vi "8-Tap 8-bit Camera with DRAM Modified (FPGA).vi"() -> ()   [LabVIEW 2013]
doc: "This is the FPGA VI for the 10-Tap 8-Bit Camera with DRAM example. This example demonstrates how to acquire images from a 10-tap, 8-bit, extended configuration, Camera Link camera and transfer the images to the host. This example supports area scan and line scan cameras for both continuous and finite acquisitions.\n\nThis example also demonstrates the use of DRAM as a frame buffer for very high speed acquisitions. Data packing and flow-control are also employed to maximize use of the available DRAM and FIFOs in terms of both memory space and performance.\n\nAdditionally, the example demonstrates the serial server, which allows third-party camera configuration utilities to communicate with the camera using the Camera Link serial interface while this VI is running."
uses:
  Common/CL Signal Mapping.ctl
  Common/CL Configuration.ctl
  <vilib>/Platform/TimedLoop/XDataNode/timing_clust.ctl
  <vilib>/Platform/TimedLoop/XDataNode/nitl_modes.ctl
  <vilib>/Platform/TimedLoop/XDataNode/wakeup.ctl
  <vilib>/rvi/Emulation/niFpgaSctlEmulationGetInTimedLoop.vi
  <vilib>/rvi/Emulation/niFpgaEmulationReportErrorSimple.vi
  <vilib>/rvi/eio/common/nirviEmuTemplateMethod_errors.vi
  <vilib>/rvi/Emulation/niFpgaGetClockAttributes.vi
  <vilib>/rvi/Emulation/niFpgaCriticalErrorInLSC.vi
  Common/CL Data to Pixels/8 Tap 8-Bit.vi
  <vilib>/rvi/FIFO/Fifo_Resource/nirvififoEmulationWriteFpgaImpl.vi
  <vilib>/rvi/DataTransferAndStorage/Container/Common/niFpgaContainerGetUniqueNameForEmu.vi
  <vilib>/rvi/FIFO/Fifo_Resource/nirvififoEmulationGetNumberOfElementsToReadFpgaImpl.vi
  <vilib>/rvi/FIFO/Fifo_Resource/nirvififoEmulationReadFpgaImpl.vi
  <vilib>/rvi/interface/RandomDataEmulation/nirviRandomDataFPGAFIFO.vi
  <vilib>/rvi/interface/RandomDataEmulation/niFpgaRandomDataHandleErrors.vi
  <vilib>/rvi/Emulation/niFpgaProcessEmulError.vi
  <vilib>/Platform/TimedLoop/XDataNode/XDataNode.xnode
  <vilib>/eio/EIONode/EIONode.xnode
  <vilib>/rvi/DataTransferAndStorage/Container/XNode/niFpgaContainer.xnode
  <vilib>/rvi/FIFO/Fifo_Resource/nirvififoEmulationWrite.vi
  <vilib>/rvi/FIFO/Fifo_Resource/nirvififoEmulationGetNumberOfElementsToRead.vi
  <vilib>/rvi/FIFO/Fifo_Resource/nirvififoEmulationRead.vi
  <vilib>/rvi/interface/RandomDataEmulation/nirviRandomDataFpgaReadWriteTemplate.vi
  <vilib>/Platform/TimedLoop/XDataNode/XDNodeRunTimeDep.lvlib
panel:
  out "DMA Full?":bool
  in  "CL Config.Configuration":T1=enum."Full"
  in  "CL Config.Signal Mapping":T2
  in  "CL Config.Line Scan":bool
  in  "CL Config.DVAL Active High":bool=TRUE
  in  "CL Config.LVAL Active High":bool=TRUE
  in  "CL Config.FVAL Active High":bool=TRUE
  in  "CL Config.Spare Active High":bool=TRUE
  in  "Acq Control.Line Scan Height":u32
  in  "Acq Control.Frames To Acq":u32
  in  "Acq Control.Acquire":bool
  in  "Acq Control.Cancel Acq":bool
  in  "Acq Control.Ignore DVAL":bool
  in  "Acq Control.Initialize":bool
  out "Acq Status.Acq In Progress":bool
  out "Acq Status.Clocks Per Line":u32
  out "Acq Status.Frames Acq'd":u32
  out "Acq Status.Lines Per Frame":u32
  out "Acq Status.DMA Write Timeout":bool
  out "Acq Status.Initialized":bool
  in  "UART.Baud Rate":u8
  in  "UART.Transmit":bool
  in  "UART.Tx Data":u8[](array[numeric])=[0, 0, 0, 0, 0, 0, 0, 0, 0, 0] format="%02x"
  in  "UART.Set Baud Rate":bool
  in  "UART.Byte Mode":bool=TRUE
  out "UART.Rx Ready":bool
  out "UART.Break Indicator":bool
  out "UART.Framing Error":bool
  out "UART.Overrun Error":bool
  out "UART.Tx Ready":bool
  out "UART.Rx Data":u8 format="%02x"
  in  "UART.Receive":bool
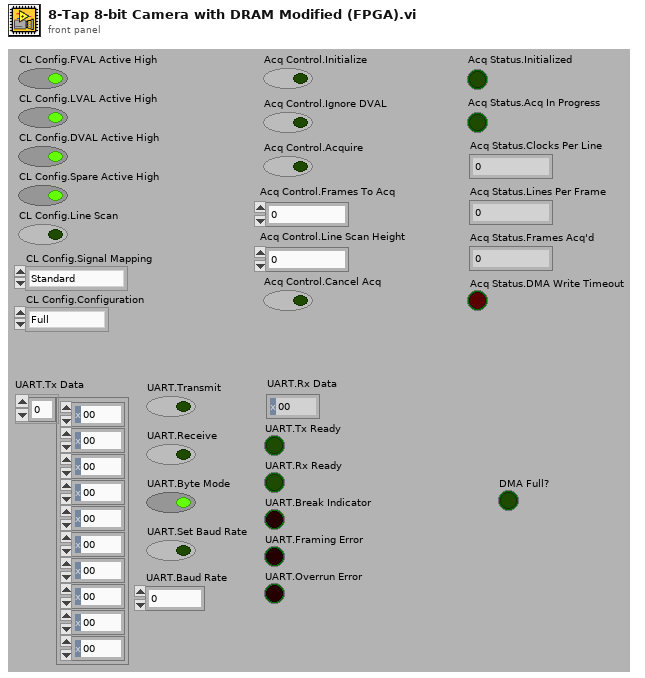
[diagram p1: front panel]
types:
  T1 = typedef "CL Configuration.ctl" = enum8{"Base", "Medium", "Full"}
  T2 = typedef "CL Signal Mapping.ctl" = enum8{"Standard", "Basler 10-tap", "Vosskühler 10-tap"}
  T3 = typedef "XDNodeRunTimeDep.lvlib/timing_clust.ctl" = cluster{"Expected End [f-1]":u64, "Actual End [f-1]":u64, "Finished Late? [f-1]":bool, "Expected End [i-1]":u64, "Actual End [i-1]":u64, "Finished Late? [i-1]":bool, "Expected Start [i]":u64, "Actual Start [i]":u64, "Expected Start [f]":u64, "Actual Start [f]":u64, "Source Name":string, "Structure Name":string, "Period":i64, "Deadline":i64, "Offset":i64, "Start":i64, "Priority":i32, "Timeout":i32, "Mode":T4, "Wakeup Reason":T5, "Error":errorcluster, "Source Type":string, "Secondary Source Type":string, "Global End Time":u64, "Global Start Time":u64, "Frame Duration":u64, "Iteration Duration":u64, "Assigned CPU":i32, "I/O Scan Engine Mode":u32}
  T4 = typedef "XDNodeRunTimeDep.lvlib/nitl_modes.ctl" = enum32{"No Change", "Process missed periods, maintain original phase", "Discard missed periods, maintain original phase", "Process missed periods, ignore original phase", "Discard missed periods, ignore original phase"}
  T5 = typedef "XDNodeRunTimeDep.lvlib/wakeup.ctl" = enum32{"Normal", "Aborted", "Asynchronous wakeup", "Timing source error", "Timed loop error", "Timeout"}
  T6 = cluster{"Enables Valid":bool, "Frame Valid":bool, "Line Valid":bool, "Data Valid":bool}
  T7 = cluster{"Pixel 0":u8, "Pixel 1":u8, "Pixel 2":u8, "Pixel 3":u8, "Pixel 4":u8, "Pixel 5":u8, "Pixel 6":u8, "Pixel 7":u8}
  T8 = cluster{"Tx Data":u8[], "Transmit":bool, "Receive":bool, "Byte Mode":bool, "Set Baud Rate":bool, "Baud Rate":u8}
  T9 = cluster{"Rx Data":u8, "Turn Off Transmit":bool, "Turn Off Receive":bool, "Turn Off Set Baud Rate":bool, "Tx Ready":bool, "Rx Ready":bool, "Break Indicator":bool, "Framing Error":bool, "Overrun Error":bool}
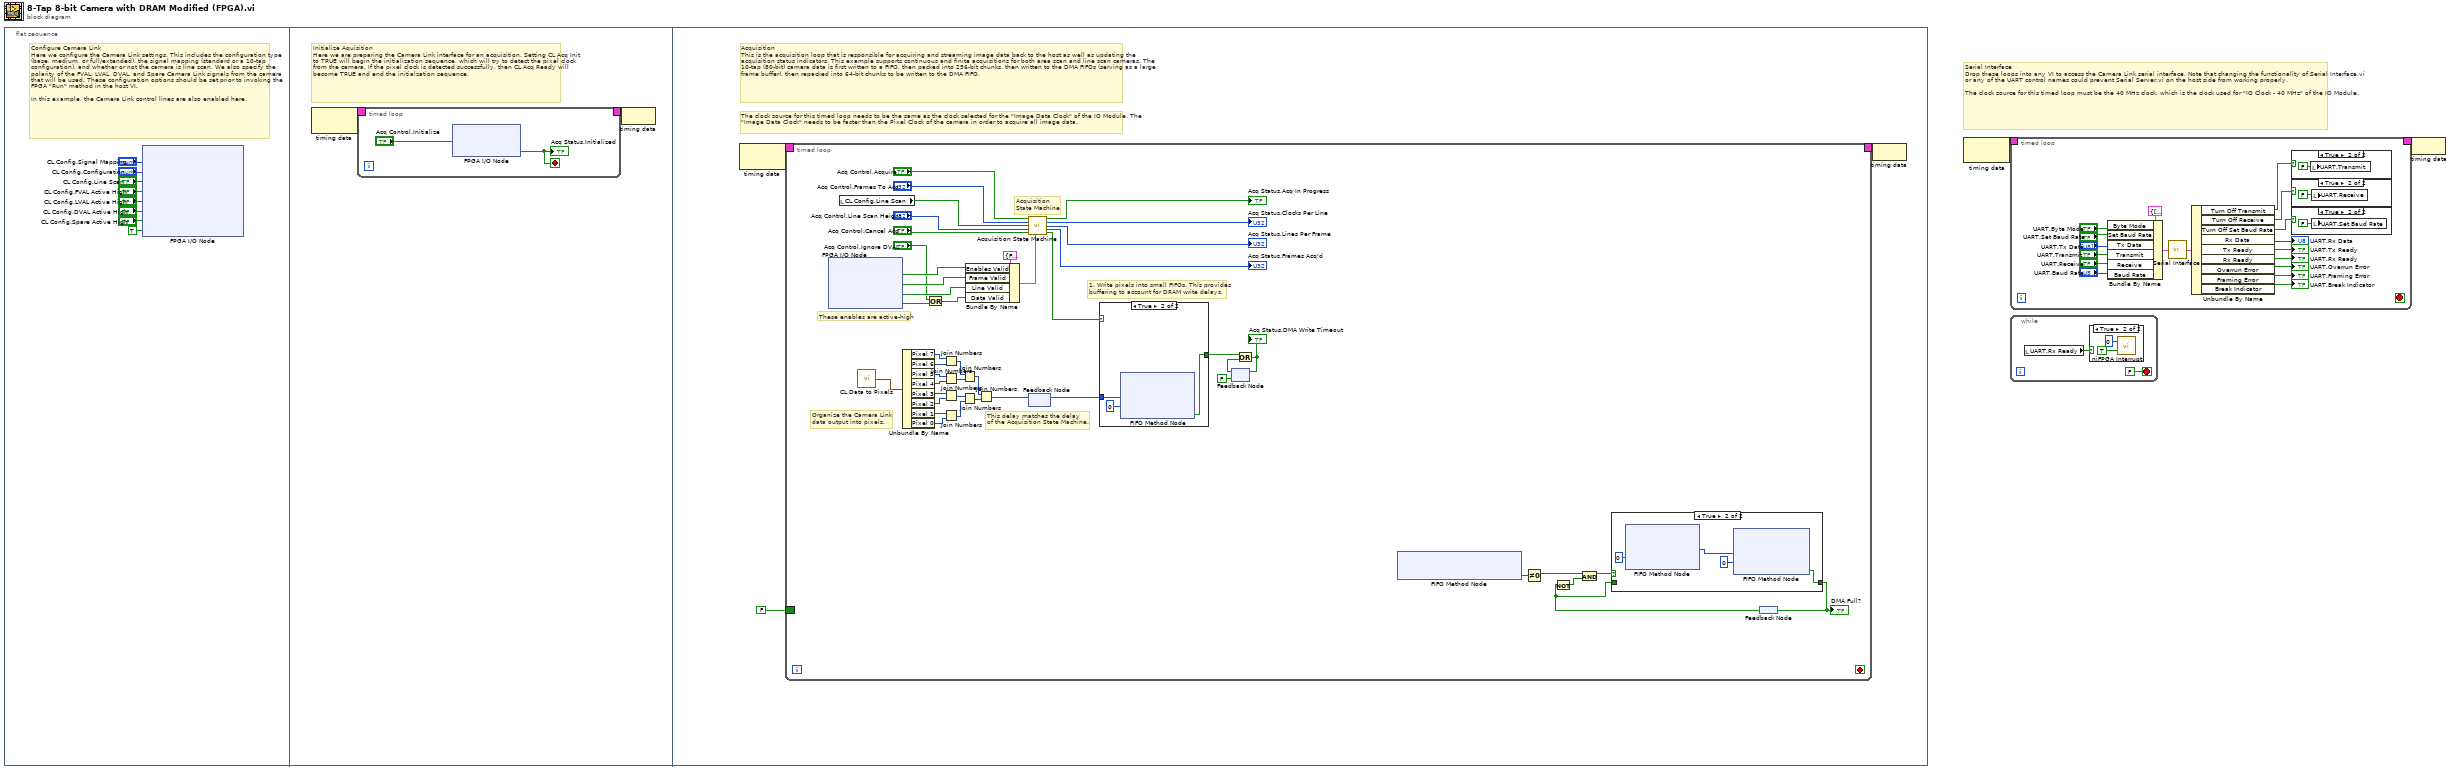
[diagram p0: block diagram]
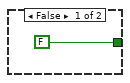
[diagram p7: hidden frame]
diagram:
  # "Serial Interface\nDrop these loops into any VI to access the Camera Link serial interface. Note that changing the functionality of Serial Interface.vi or any of the UART control names could prevent Serial Server.vi on the host side from working properly.\n\nThe clock source for this timed loop must be the 40 MHz clock, which is the clock used for \"IO Clock - 40 MHz\" of the IO Module."
  n1 = flat-sequence {
    frame #0 {
      # "Configure Camera Link\nHere we configure the Camera Link settings. This includes the configuration type (base, medium, or full/extended), the signal mapping (standard or a 10-tap configuration), and whether or not the camera is line scan. We also specify the polarity of the FVAL, LVAL, DVAL, and Spare Camera Link signals from the camera that will be used. These configuration options should be set prior to invoking the FPGA \"Run\" method in the host VI.\n\nIn this example, the Camera Link control lines are also enabled here."
      n2 = xnode "FPGA I/O Node"("CL Set Signal Mapping"="CL Config.Signal Mapping", "CL Set Configuration"="CL Config.Configuration", "CL Set Line Scan"="CL Config.Line Scan", "CL Set FVAL Active High"="CL Config.FVAL Active High", "CL Set LVAL Active High"="CL Config.LVAL Active High", "CL Set DVAL Active High"="CL Config.DVAL Active High", "CL Set Spare Active High"="CL Config.Spare Active High", "CL Control Enable"=TRUE ("IO Module\\CL Control Enable")) -> ()  [unwired: 8 in, 8 out]
    }
    frame #1 {
      # "Initialize Aquisition\nHere we are preparing the Camera Link interface for an acquisition. Setting CL Acq Init to TRUE will begin the initialization sequence, which will try to detect the pixel clock from the camera. If the pixel clock is detected successfully, then CL Acq Ready will become TRUE and end the initialzation sequence."
      n3 = node-c288() -> (w12:T3)  [unwired: 1 out]
      n4 = timed-loop {
        timing: w12 -> [_]
        timing-out: [_] -> w11
        stop <- w13 stop-if-true
        n5 = xnode "FPGA I/O Node"("CL Acq Init"="Acq Control.Initialize") -> ("CL Acq Ready"=w13:bool)  [unwired: 2 in, 2 out]
        "Acq Status.Initialized" <- w13
      }
      n6 = node-c288(w11) -> ()
    }
    frame #2 {
      # "The clock source for this timed loop needs to be the same as the clock selected for the \"Image Data Clock\" of the IO Module. The \"Image Data Clock\" needs to be faster than the Pixel Clock of the camera in order to acquire all image data."
      # "Acquisition\nThis is the acquisition loop that is responsible for acquiring and streaming image data back to the host as well as updating the acquisition status indicators. This example supports continuous and finite acquisitions for both area scan and line scan cameras. The 10-tap (80-bit) camera data is first written to a FIFO, then packed into 256-bit chunks, then written to the DMA FIFOs (serving as a large frame buffer), then repacked into 64-bit chunks to be written to the DMA FIFO."
      n7 = node-c288() -> (w21:T3)  [unwired: 1 in]
      n8 = timed-loop {
        timing: w21 -> [_]
        timing-out: [_] -> w20
        border: FALSE ("Timed Out?") -> [_]
        stop <- _ stop-if-true
        # "1. Write pixels into small FIFOs. This provides\nbuffering to account for DRAM write delays."
        # "Organize the Camera Link\ndata output into pixels."
        # "These enables are active-high"
        # "This delay matches the delay\nof the Acquisition State Machine."
        # "Acquisition\nState Machine"
        n9 = xnode "FPGA I/O Node"() -> ("CL Output Valid"=w52:bool, "CL Frame Valid"=w51:bool, "CL Line Valid"=w50:bool, "CL Data Valid"=w47:bool)  [unwired: 4 in, 4 out]
        n10 = local read "CL Config.Line Scan"() -> (w44:bool)
        n11 = call-poly "CL Data to Pixels.vi"() -> ("Pixels"=w66:T7)  [unwired: 1 in]
        n12 = Unbundle By Name(w66) -> ("Pixel 7"=w42:u8, "Pixel 6"=w41:u8, "Pixel 5"=w40:u8, "Pixel 4"=w39:u8, "Pixel 3"=w38:u8, "Pixel 2"=w37:u8, "Pixel 1"=w36:u8, "Pixel 0"=w35:u8)
        n13 = Or(x="Acq Control.Ignore DVAL", y=w47) -> (x .or. y?=w46:bool)
        n14 = Join Numbers(hi=w42, lo=w41) -> ((hi.lo)=w33:u16)
        n15 = Join Numbers(hi=w40, lo=w39) -> ((hi.lo)=w32:u16)
        n16 = Join Numbers(hi=w38, lo=w37) -> ((hi.lo)=w31:u16)
        n17 = Join Numbers(hi=w36, lo=w35) -> ((hi.lo)=w34:u16)
        n18 = Join Numbers(hi=w33, lo=w32) -> ((hi.lo)=w30:u32)
        n19 = Join Numbers(hi=w31, lo=w34) -> ((hi.lo)=w29:u32)
        n20 = Bundle By Name(cluster=T6 {"Enables Valid"=FALSE, "Frame Valid"=FALSE, "Line Valid"=FALSE, "Data Valid"=FALSE} ("Enables"), "Enables Valid"=w52, "Frame Valid"=w51, "Line Valid"=w50, "Data Valid"=w46) -> (w49:T6)
        n21 = Join Numbers(hi=w30, lo=w29) -> ((hi.lo)=w28:u64)
        n22 = call "Acquisition State Machine.vi"("Acquire"="Acq Control.Acquire", "Frames to Acquire"="Acq Control.Frames To Acq", "Line Scan"=w44, "Line Scan Height"="Acq Control.Line Scan Height", "Cancel Acq"="Acq Control.Cancel Acq", "Enables"=w49) -> ("Acq In Progress"=→"Acq Status.Acq In Progress":bool, "Num Clocks Per Line"=→"Acq Status.Clocks Per Line":u32, "Num Lines Per Frame"=→"Acq Status.Lines Per Frame":u32, "Num Frames Acq'd"=→"Acq Status.Frames Acq'd":u32, "Capture Cycle"=w64:bool)  [unwired: 4 in, 1 out]
        n23 = feedback-in #1(w28) -> ()
        n24 = feedback #1() -> (w65:u64)  [unwired: 1 in]
        n25 = case shown="True" w64 {
          tunnel: [FALSE ("Timed Out?") w74] -> w62
          tunnel: w65 -> [_ w75]
          frame False {
          }
          frame True {
            n26 = xnode ("FIFO Method Node")("Element"=w75, "Timeout"=0) -> ("Timed Out?"=w74:bool)  [unwired: 1 in, 1 out]
          }
        }
        n27 = feedback #2(FALSE) -> (w61:bool)
        n28 = Or(x=w62, y=w61) -> (x .or. y?=w60:bool)
        "Acq Status.DMA Write Timeout" <- w60
        n29 = feedback-in #2(w60) -> ()
        n30 = xnode ("FIFO Method Node")() -> ("Number of Elements to Read"=w27:u32)  [unwired: 1 in, 1 out]
        n31 = Not Equal To 0?(x=w27) -> (x != 0?=w22:bool)
        n32 = feedback #3() -> (w23:bool)
        n33 = Not(x=w23) -> (.not. x?=w24:bool)
        n34 = And(x=w22, y=w24) -> (x .and. y?=w25:bool)
        n35 = case shown="True" w25 {
          tunnel: [w67 w70] -> w26
          tunnel: w23 -> [w67 _]
          frame False {
          }
          frame True {
            n36 = xnode ("FIFO Method Node")("Timeout"=0) -> ("Element"=w68:u64)  [unwired: 1 in, 2 out]
            n37 = xnode ("FIFO Method Node")("Element"=w68, "Timeout"=0) -> ("Timed Out?"=w70:bool)  [unwired: 1 in, 1 out]
          }
        }
        "DMA Full?" <- w26
        n38 = feedback-in #3(w26) -> ()
      }
      n39 = node-c288(w20) -> ()
    }
  }
  n40 = node-c288() -> (w2:T3)  [unwired: 1 out]
  n41 = timed-loop {
    timing: w2 -> [_]
    timing-out: [_] -> w1
    stop <- _ stop-if-true
    n42 = Bundle By Name(cluster=T8 {"Tx Data"=[0, 0, 0, 0, 0, 0, 0, 0, 0, 0], "Transmit"=FALSE, "Receive"=FALSE, "Byte Mode"=TRUE, "Set Baud Rate"=FALSE, "Baud Rate"=0} ("UART Inputs"), "Byte Mode"="UART.Byte Mode", "Set Baud Rate"="UART.Set Baud Rate", "Tx Data"="UART.Tx Data", "Transmit"="UART.Transmit", "Receive"="UART.Receive", "Baud Rate"="UART.Baud Rate") -> (w80:T8)
    n43 = call "Serial Interface.vi"("UART Inputs"=w80) -> ("UART Outputs"=w92:T9)
    n44 = Unbundle By Name(w92) -> ("Turn Off Transmit"=w85:bool, "Turn Off Receive"=w86:bool, "Turn Off Set Baud Rate"=w82:bool, "Rx Data"=→"UART.Rx Data":u8, "Tx Ready"=→"UART.Tx Ready":bool, "Rx Ready"=→"UART.Rx Ready":bool, "Overrun Error"=→"UART.Overrun Error":bool, "Framing Error"=→"UART.Framing Error":bool, "Break Indicator"=→"UART.Break Indicator":bool)
    n45 = case shown="True" w85 {
      frame False {
      }
      frame True {
        n46 = local write "UART.Transmit"(FALSE ("UART.Transmit")) -> ()
      }
    }
    n47 = case shown="True" w86 {
      frame False {
      }
      frame True {
        n48 = local write "UART.Receive"(FALSE ("UART.Receive")) -> ()
      }
    }
    n49 = case shown="True" w82 {
      frame False {
      }
      frame True {
        n50 = local write "UART.Set Baud Rate"(FALSE ("UART.Receive")) -> ()
      }
    }
  }
  n51 = while {
    stop <- FALSE stop-if-true
    n52 = local read "UART.Rx Ready"() -> (w104:bool)
    n53 = case shown="True" w104 {
      frame False {
      }
      frame True {
        n54 = call <vilib>:"niFPGA Interrupt.vi"("Wait Until Cleared (F)"=TRUE ("Wait Until Cleared"), "IRQ Number (0)"=u8 0 ("IRQ Number")) -> ()  [unwired: 1 in]
      }
    }
  }
  n55 = node-c288(w1) -> ()
